vi "PQasyncQueryCommand.vi"(9 "query":string, 11 "conn":u64) -> (0 "PQresultErrorMessage":string, 1 "PQresultStatus":T1(ring), 2 "PGresult":u64, 3 "PQsendQuery":u64)   [LabVIEW 2019, in "libpqutility64.lvlib"]
doc: "Asynchronours Querry Commando Execution\nSee PostgreSQL c-lib doku for further information."
uses:
  libpqutility64.lvlib
  libpqlv64/libpqlv64.lvlib
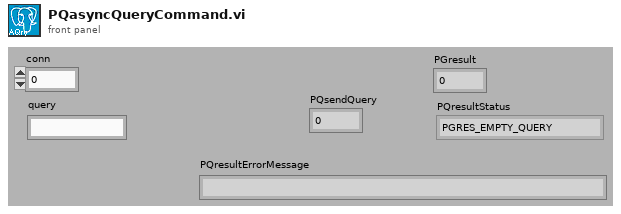
[diagram p1: front panel]
types:
  T1 = enum32{"PGRES_EMPTY_QUERY", "PGRES_COMMAND_OK", "PGRES_TUPLES_OK", "PGRES_COPY_OUT", "PGRES_COPY_IN", "PGRES_BAD_RESPONSE", "PGRES_NONFATAL_ERROR", "PGRES_FATAL_ERROR"}
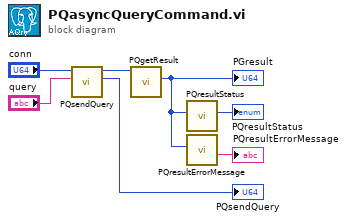
[diagram p0: block diagram]
diagram:
  n1 = call "PQsendQuery.vi"("query"="query", "conn"="conn") -> ("PQsendQuery"=→"PQsendQuery":i64, "conn_out"=w1:u64)  [unwired: 7 in, 1 out]
  n2 = call "PQgetResult.vi"("conn"=w1) -> ("PGresult"=w5:u64)  [unwired: 8 in, 2 out]
  "PGresult" <- w5
  n3 = call "PQresultStatus.vi"("res"=w5) -> ("res out"=→"PQresultStatus":u64)  [unwired: 8 in, 2 out]
  n4 = call "PQresultErrorMessage.vi"("res"=w5) -> ("PQresultErrorMessage"=→"PQresultErrorMessage":string)  [unwired: 8 in, 2 out]
